vi "Create User Events.vi"(8 "error in (no error)":errorcluster) -> (0 "error out":errorcluster, 2 "User Events":T1, 3 "User Events Registration Refnum":refnum<event-registration>)   [LabVIEW 2014, in "User Events.lvlib"]
doc: "Create a boolean user event that will be used to stop the event loop from the message handling loop."
uses:
  User Events.lvlib
  User Events.ctl
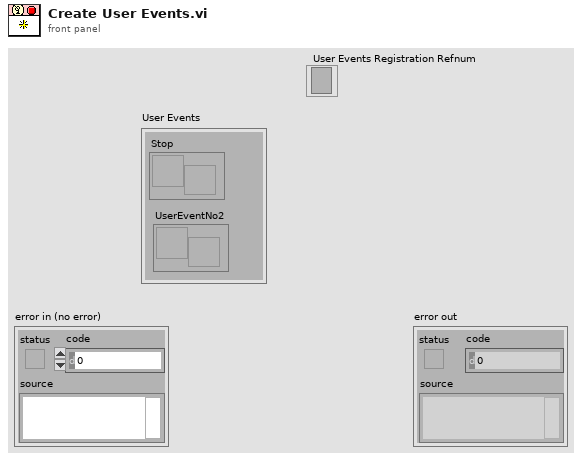
[diagram p1: front panel]
types:
  T1 = typedef "User Events.lvlib/User Events.ctl" = cluster{"Stop":refnum<user-event>, "UserEventNo2":refnum<user-event>}
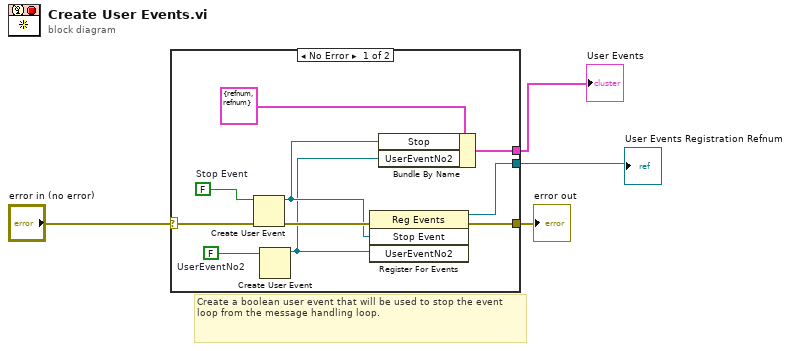
[diagram p0: block diagram]
diagram:
  # "Create a boolean user event that will be used to stop the event loop from the message handling loop."
  n1 = case shown="No Error" "error in (no error)" {
    selector: "error in (no error)" -> [w10 w15]
    tunnel: [w14 _] -> w4
    tunnel: [w11 w15] -> w3
    tunnel: [w5 _] -> w1
    frame No Error {
      w9 = FALSE  # UserEventNo2
      w13 = FALSE  # Stop Event
      n2 = Create User Event(user event datatype=w13, error in=w10) -> (user event=w7:refnum<user-event>, error out=w12:errorcluster)
      n3 = Create User Event(user event datatype=w9) -> (user event=w6:refnum<user-event>)  [unwired: 1 in, 1 out]
      n4 = register-events(error in=w12, w7, w6) -> (reference out=w14:refnum<event-registration>, error out=w11:errorcluster)  [unwired: 1 in]
      n5 = Bundle By Name(cluster=T1 {"Stop"=refnum, "UserEventNo2"=refnum} ("User Events 2"), "Stop"=w7, "UserEventNo2"=w6) -> (w5:T1)
    }
    frame Error {
    }
  }
  "error out" <- w3
  "User Events" <- w1
  "User Events Registration Refnum" <- w4
